vi "Measurement Logic.vi"() -> ()   [LabVIEW 2021, in "Table and Multicolumn Listbox.lvlib"]
uses:
  Table and Multicolumn Listbox.lvlib
  Measurement Configuration.ctl
  Measurement Results.ctl
  <vilib>/MeasurementLink/MeasurementLink Measurement Server/Measure Call Context/Measure Call Context.lvclass
panel:
  out "measure call context out":refnum<class "Measure Call Context.lvclass">
  in  "measure call context in":refnum<class "Measure Call Context.lvclass">
  out "measurement results":T1
  in  "measurement configuration":T2
  out "error out":errorcluster
  in  "error in":errorcluster
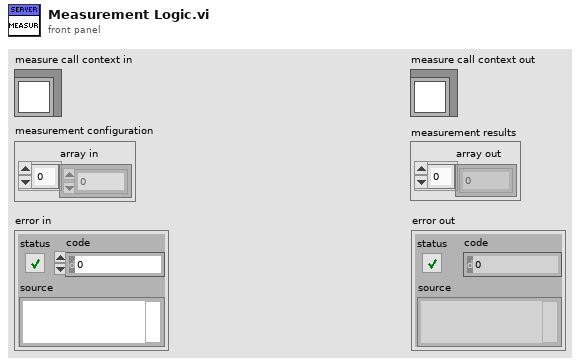
[diagram p1: front panel]
types:
  T1 = typedef "Table and Multicolumn Listbox.lvlib/Measurement Results.ctl" = cluster{"array out":dbl[]}
  T2 = typedef "Table and Multicolumn Listbox.lvlib/Measurement Configuration.ctl" = cluster{"array in":dbl[]}
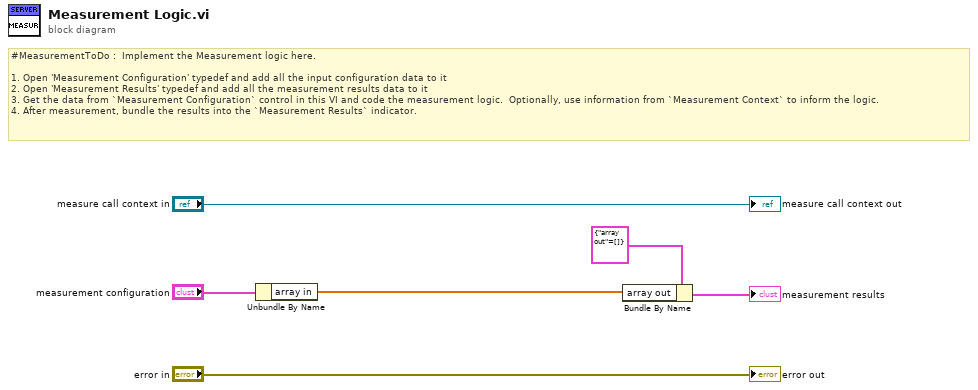
[diagram p0: block diagram]
diagram:
  # "#MeasurementToDo :  Implement the Measurement logic here.\n\n1. Open 'Measurement Configuration' typedef and add all the input configuration data to it\n2. Open 'Measurement Results' typedef and add all the measurement results data to it\n3. Get the data from `Measurement Configuration` control in this VI and code the measurement logic.  Optionally, use information from `Measurement Context` to inform the logic.\n4. After measurement, bundle the results into the `Measurement Results` indicator."
  n1 = Unbundle By Name("measurement configuration") -> ("array in"=w3:dbl[])
  n2 = Bundle By Name(cluster=T1 {"array out"=[]} ("Measurement Results"), "array out"=w3) -> (→"measurement results":T1)
  "error out" <- "error in"
  "measure call context out" <- "measure call context in"
